vi "read_attributes.vi"(8 "error in (no error)":errorcluster, 11 "LinearSVC in":refnum<class "LinearSVC.lvclass">) -> (0 "error out":errorcluster, 2 "attributes":T1, 3 "LinearSVC out":refnum<class "LinearSVC.lvclass">)   [LabVIEW 2020, in "LinearSVC.lvclass"]
uses:
  LinearSVC.lvclass
  Controls/linear_svc_attributes.ctl
  LinearSVC.lvclass/LinearSVC.ctl
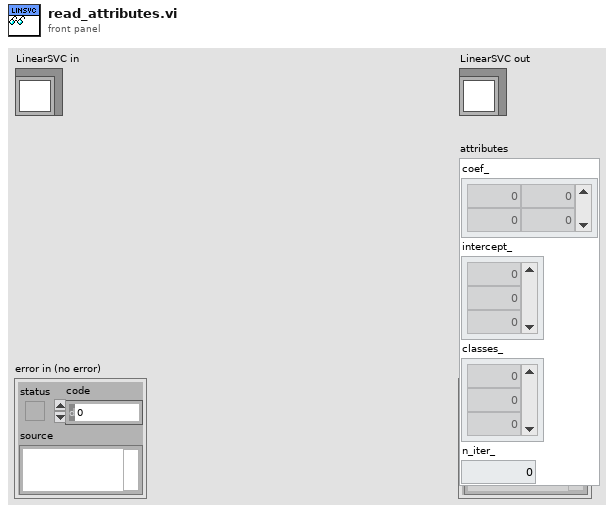
[diagram p1: front panel]
types:
  T1 = typedef "linear_svc_attributes.ctl" = cluster{"coef_":dbl[][], "intercept_":dbl[], "classes_":dbl[], "n_iter_":dbl}
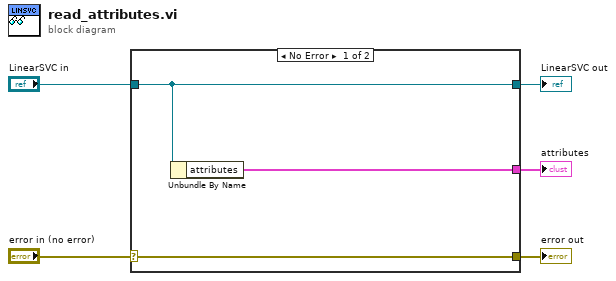
[diagram p0: block diagram]
diagram:
  n1 = case shown="No Error" "error in (no error)" {
    selector: "error in (no error)" -> [w8 w9]
    tunnel: [w8 w9] -> w4
    tunnel: [w7 w10] -> w2
    tunnel: "LinearSVC in" -> [w7 w10]
    tunnel: [w6 _] -> w1
    frame No Error {
      n2 = Unbundle By Name(w7) -> ("attributes"=w6:T1)
    }
    frame Error {
    }
  }
  "error out" <- w4
  "LinearSVC out" <- w2
  "attributes" <- w1
